vi "test.vi"() -> ()   [LabVIEW 2019]
uses:
  <vilib>/FPGAPlugInAG/cRIO-9042/niLvFpga_Open_cRIO-9042.vi
  <vilib>/rvi/interface/common/dynamic/niFpgaDynamicAddResources.vi
  <vilib>/FPGAPlugInAG/Dynamic/niLvFpga_Run_Dynamic.vi
  <vilib>/Utility/error.llb/Error Cluster From Error Code.vi
  <vilib>/rvi/errors/niLvFpgaAdjustHostInterfaceError.vi
  <vilib>/FPGAPlugInAG/Dynamic/niLvFpga_Close_Dynamic.vi
  <vilib>/rvi/interface/nirviOpenFPGA/nirviOpenFPGA.xnode
  FPGA Bitfiles/auxtelmaindomeco_FPGATarget2_fpga_Pb8v0YOByPU.lvbitx
  <vilib>/rvi/interface/nirviMethod/nirviMethod.xnode
  <vilib>/rvi/interface/nirviReadWriteControl/nirviReadWriteControl.xnode
  <vilib>/rvi/interface/nirviCloseFPGA/nirviCloseFPGA.xnode
  NiFpgaLv.dll
  <vilib>/rvi/interface/Simulation/niFpgaSimulationCallBeginRW.vi
  <vilib>/NI_Real-Time Target Support.lvlib
panel:
  out "Chassis Temperature":i16
  out "config out":T1
  out "homing wait counter":u32
  out "buttons":T2
  out "led":bool
  out "exit?":bool
  out "homing?":bool
  out "cmd":i8
  out "cmd request":i8
  out "rev dly counter":u32
  out "home sensor":bool
  out "env sensor":bool
  out "az to counter":u32
  out "cloud to counter":u32
  out "cloud?":bool
  out "enc status":u16
  out "sub mode":u8
  out "mode":u8
  out "az pos [deg]":dbl
  out "az enc counts":u64
  out "errors":T3
  out "error?":bool
  out "az last rotation":enum16{"none", "forward", "reverse"}(ring)
  out "rs":bool
  in  "az pos req [deg]":dbl min=0.0 max=360.0 format="%#_13g"
  in  "shutdown":bool
  in  "emergency stop":bool
  in  "mode request":enum16{"stop", "home", "position", "center"}(ring)
  in  "reset":bool
  in  "config":T1={"io.cloud-enable"=FALSE, "io.encoder-negate"=FALSE, "io.encoder-ref"=79895940197, "io.encoder-step"=4018143232, "io.home-pos"=0.0, "sm.az-timeout (ms)"=120000, "sm.encoder-no-error"=1025, "sm.main-pos-hs-thres"=0.013888888992369175, "sm.main-pos-tol"=0.00138888880610466, "sm.cloud-timeout (ms)"=100000, "sm.rev-dly (ms)"=4000, "io.encoder-center"=68719476735, "sm-main-center-hs-thres"=55807545, "sm-main-center-tol"=5580754}
  in  "stop":bool
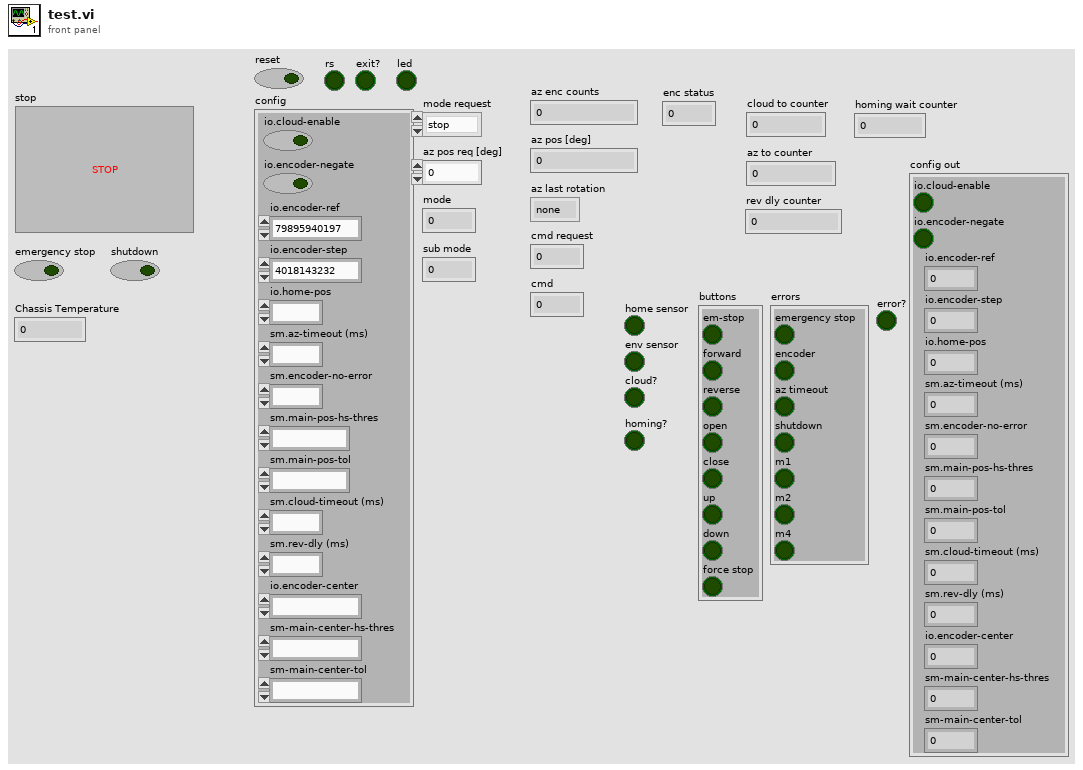
[diagram p1: front panel]
types:
  T1 = cluster{"io.cloud-enable":bool, "io.encoder-negate":bool, "io.encoder-ref":u64, "io.encoder-step":u64, "io.home-pos":fxp<+/-,32,2>, "sm.az-timeout (ms)":u32, "sm.encoder-no-error":u16, "sm.main-pos-hs-thres":fxp<+/-,32,2>, "sm.main-pos-tol":fxp<+/-,32,2>, "sm.cloud-timeout (ms)":u32, "sm.rev-dly (ms)":u32, "io.encoder-center":u64, "sm-main-center-hs-thres":u64, "sm-main-center-tol":u64}
  T2 = cluster{"em-stop":bool, "forward":bool, "reverse":bool, "open":bool, "close":bool, "up":bool, "down":bool, "force stop":bool}
  T3 = cluster{"emergency stop":bool, "encoder":bool, "az timeout":bool, "shutdown":bool, "m1":bool, "m2":bool, "m4":bool}
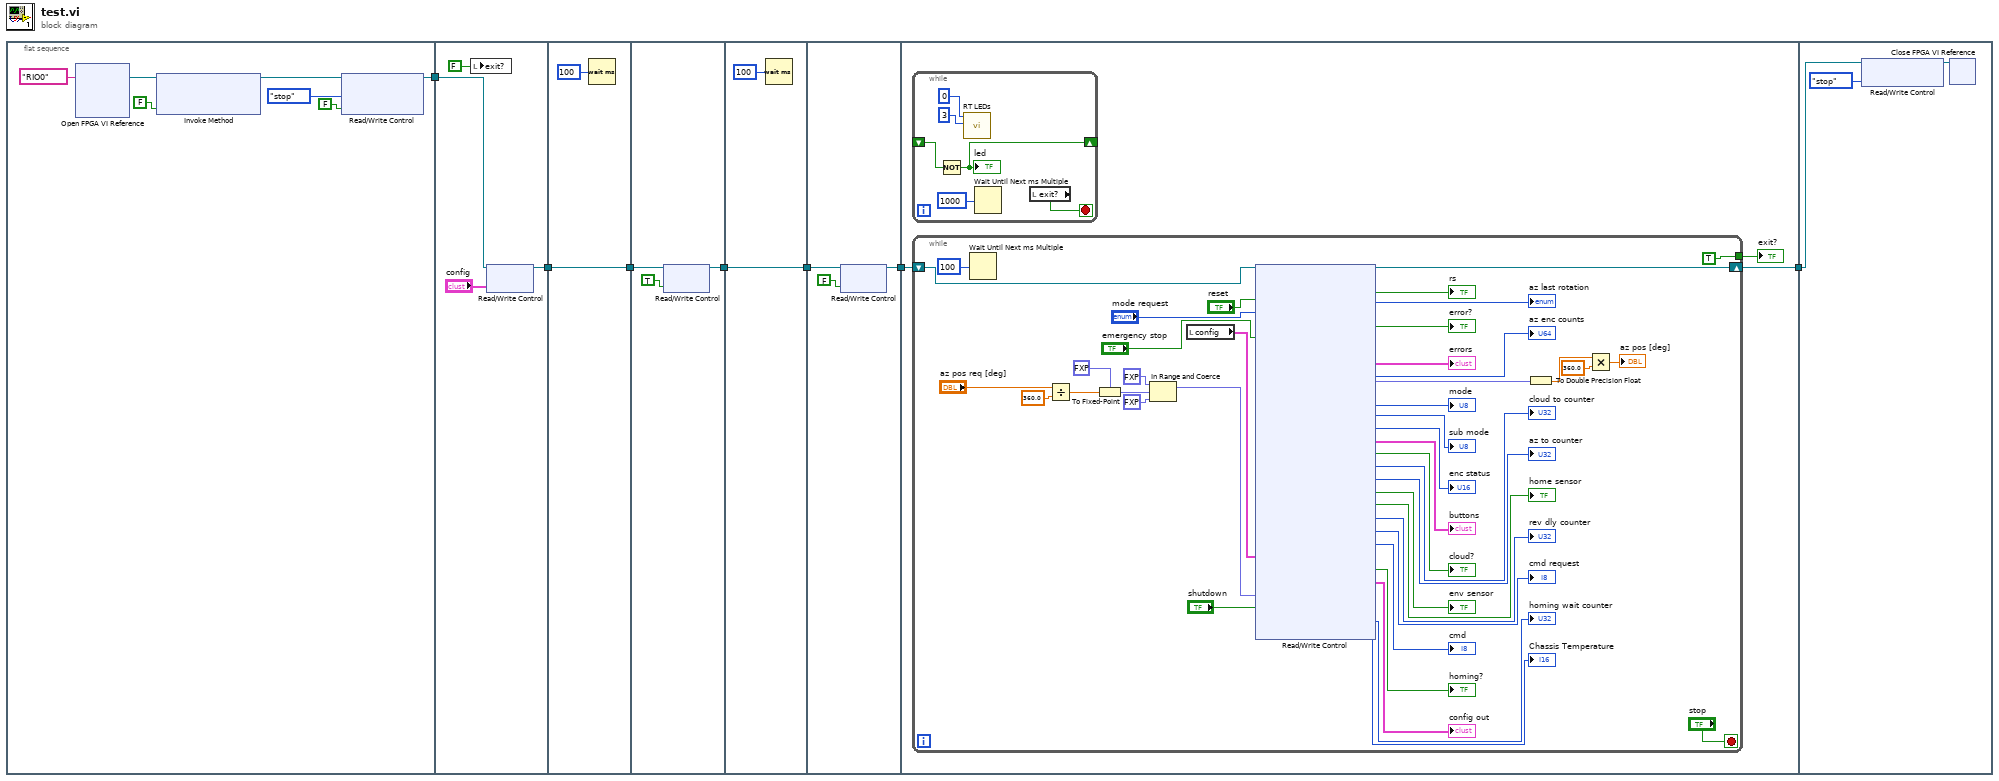
[diagram p0: block diagram]
diagram:
  n1 = flat-sequence {
    tunnel: [w12] -> w3
    tunnel: w3 -> [w18]
    tunnel: [w16] -> w2
    tunnel: w2 -> [w20]
    tunnel: [w20] -> w1
    tunnel: [w22] -> w6
    tunnel: w1 -> [w21]
    tunnel: w6 -> [w24]
    tunnel: [w24] -> w5
    tunnel: w5 -> [w27]
    tunnel: [w26] -> w4
    tunnel: [w31] -> w7
    tunnel: w4 -> [w30]
    tunnel: w7 -> [w82]
    frame #0 {
      n2 = xnode "Open FPGA VI Reference"("resource name"=tag "RIO0") -> ("FPGA VI Reference Out"=w9:refnum<k20>)  [unwired: 1 in, 1 out]
      n3 = xnode "Invoke Method"("FPGA VI Reference In"=w9, "Wait Until Done (F)"=FALSE) -> ("FPGA VI Reference Out"=w14:refnum<k20>)  [unwired: 1 in, 1 out]
      n4 = xnode "Read/Write Control"("FPGA VI Reference In"=w14, "mode request"=enum16{"stop", "home", "position"}."stop", "reset"=FALSE) -> ("FPGA VI Reference Out"=w12:refnum<k20>)  [unwired: 1 in, 1 out]
    }
    frame #1 {
      n5 = local write "exit?"(FALSE ("exit?")) -> ()
      n6 = xnode "Read/Write Control"("FPGA VI Reference In"=w18, "config"="config") -> ("FPGA VI Reference Out"=w16:refnum<k20>)  [unwired: 1 in, 1 out]
    }
    frame #2 {
      n7 = Wait (ms)(milliseconds to wait=u32 100) -> ()  [unwired: 1 out]
    }
    frame #3 {
      n8 = xnode "Read/Write Control"("FPGA VI Reference In"=w21, "reset"=TRUE) -> ("FPGA VI Reference Out"=w22:refnum<k20>)  [unwired: 1 in, 1 out]
    }
    frame #4 {
      n9 = Wait (ms)(milliseconds to wait=u32 100) -> ()  [unwired: 1 out]
    }
    frame #5 {
      n10 = xnode "Read/Write Control"("FPGA VI Reference In"=w27, "reset"=FALSE) -> ("FPGA VI Reference Out"=w26:refnum<k20>)  [unwired: 1 in, 1 out]
    }
    frame #6 {
      n11 = while {
        shift-right: [w32] -> _
        shift-left: _ -> [w33]
        stop <- w37 stop-if-true
        n12 = Not(x=w33) -> (.not. x?=w32:bool)
        "led" <- w32
        n13 = call <vilib>:"RT LEDs.vi"("State"=3, "LED Num"=0) -> ()  [unwired: 4 in, 2 out]
        n14 = Wait Until Next ms Multiple(millisecond multiple=u32 1000) -> ()  [unwired: 1 out]
        n15 = local read "exit?"() -> (w37:bool)
      }
      n16 = while {
        shift-right: [w63] -> w31
        shift-left: w30 -> [w78]
        tunnel: [TRUE] -> w29
        stop <- "stop" stop-if-true
        n17 = Wait Until Next ms Multiple(millisecond multiple=u32 100) -> ()  [unwired: 1 out]
        n18 = Divide(x="az pos req [deg]", y=360.0) -> (x/y=w70:dbl)
        n19 = To Fixed-Point(fixed-point type=fxp<+/-,32,2> 0.0 ("az pos req"), number=w70) -> (fixed-point=w68:fxp<+/-,32,2>)
        n20 = In Range and Coerce(upper limit=fxp<+/-,32,2> 1.0, x=w68, lower limit=fxp<+/-,32,2> 0.0) -> (coerced(x)=w65:fxp<+/-,32,2>)  [unwired: 1 out]
        n21 = local read "config"() -> (w77:T1)
        n22 = xnode "Read/Write Control"("FPGA VI Reference In"=w78, "reset"="reset", "mode request"="mode request", "emergency stop"="emergency stop", "config"=w77, "az pos req"=w65, "shutdown"="shutdown") -> ("FPGA VI Reference Out"=w63:refnum<k20>, "rs"=→"rs":bool, "az last rotation"=→"az last rotation":enum16{"none", "forward", "reverse"}, "error?"=→"error?":bool, "errors"=→"errors":T3, "az enc counts"=→"az enc counts":u64, "az pos"=w58:fxp<+/-,32,2>, "mode"=→"mode":u8, "sub mode"=→"sub mode":u8, "enc status"=→"enc status":u16, "buttons"=→"buttons":T2, "cloud?"=→"cloud?":bool, "cloud to counter"=→"cloud to counter":u32, "az to counter"=→"az to counter":u32, "env sensor"=→"env sensor":bool, "home sensor"=→"home sensor":bool, "rev dly counter"=→"rev dly counter":u32, "cmd request"=→"cmd request":i8, "cmd"=→"cmd":i8, "homing?"=→"homing?":bool, "config out"=→"config out":T1, "homing wait counter"=→"homing wait counter":u32, "Chassis Temperature"=→"Chassis Temperature":i16)  [unwired: 1 in, 1 out]
        n23 = To Double Precision Float(number=w58) -> (double precision float=w57:dbl)
        n24 = Multiply(x=w57, y=360.0) -> (x*y=→"az pos [deg]":dbl)
      }
      "exit?" <- w29
    }
    frame #7 {
      n25 = xnode "Read/Write Control"("FPGA VI Reference In"=w82, "mode request"=enum16{"stop", "home", "position"}."stop") -> ("FPGA VI Reference Out"=w83:refnum<k20>)  [unwired: 1 in, 1 out]
      n26 = xnode "Close FPGA VI Reference"("FPGA VI Reference In"=w83) -> ()  [unwired: 1 in, 1 out]
    }
  }
